vi "MoveMotor.vi"(7 "Position Mode (Absolute)":T1(ring), 8 "error in (no error)":errorcluster, 9 "Target Position (0)":i32, 10 "Axis or Vector Space":u16(ring)=1 items=["Axis 1"=1, "Axis 2"=2, "Axis 3"=3, "Axis 4"=4, "Axis 5"=5, "Axis 6"=6, "Axis 7"=7, "Axis 8"=8, "Vector Space 1"=17, "Vector Space 2"=18, "Vector Space 3"=19, "Vector Space 4"=20], 11 "Motion Bd ID":u8=1 min=1 max=32 step=1) -> (0 "error out":errorcluster, 2 "Resource Output":u16(ring) items=["Axis Control"=0, "Axis 1"=1, "Axis 2"=2, "Axis 3"=3, "Axis 4"=4, "Axis 5"=5, "Axis 6"=6, "Axis 7"=7, "Axis 8"=8, "Vector Space Control"=16, "Vector Space 1"=17, "Vector Space 2"=18, "Vector Space 3"=19, "Vector Space 4"=20, "Encoder Control"=32, "Encoder 1"=33, "Encoder 2"=34, "Encoder 3"=35, "Encoder 4"=36, "Encoder 5"=37, "Encoder 6"=38, "Encoder 7"=39, "Encoder 8"=40, "DAC Channel 1"=49, "DAC Channel 2"=50, "DAC Channel 3"=51, "DAC Channel 4"=52, "DAC Channel 5"=53, "DAC Channel 6"=54, "DAC Channel 7"=55, "DAC Channel 8"=56, "Stepper Output 1"=65, "Stepper Output 2"=66, "Stepper Output 3"=67, "Stepper Output 4"=68, "Stepper Output 5"=69, "Stepper Output 6"=70, "Stepper Output 7"=71, "Stepper Output 8"=72, "ADC Channel 1"=81, "ADC Channel 2"=82, "ADC Channel 3"=83, "ADC Channel 4"=84, "ADC Channel 5"=85, "ADC Channel 6"=86, "ADC Channel 7"=87, "ADC Channel 8"=88], 3 "Bd ID Out":u8)   [LabVIEW 2022 SP3]
uses:
  <vilib>/Motion/FlexMotion/FunctionsVIs/StartStopMotion.llb/Start Motion (8 axes).flx
  <vilib>/Motion/FlexMotion/FunctionsVIs/Trajectory.llb/Check Move Complete Status (8 axes).flx
panel:
  in  "Strict Positioning":bool
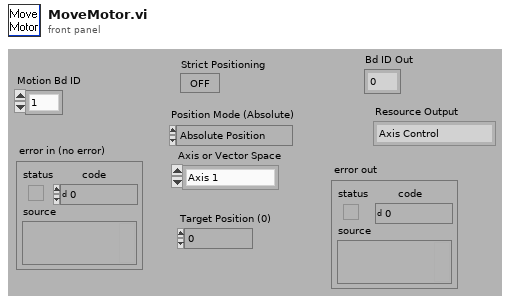
[diagram p1: front panel]
types:
  T1 = enum16{"Absolute Position", "Relative Position", "Velocity", "Relative to Cap Pos", "Modulus Position", "Absolute Contouring", "Relative Contouring"}
  T2 = typedef "Resource Out (Enum).flx" = u16
  T3 = typedef "Bd Id Out" = u8
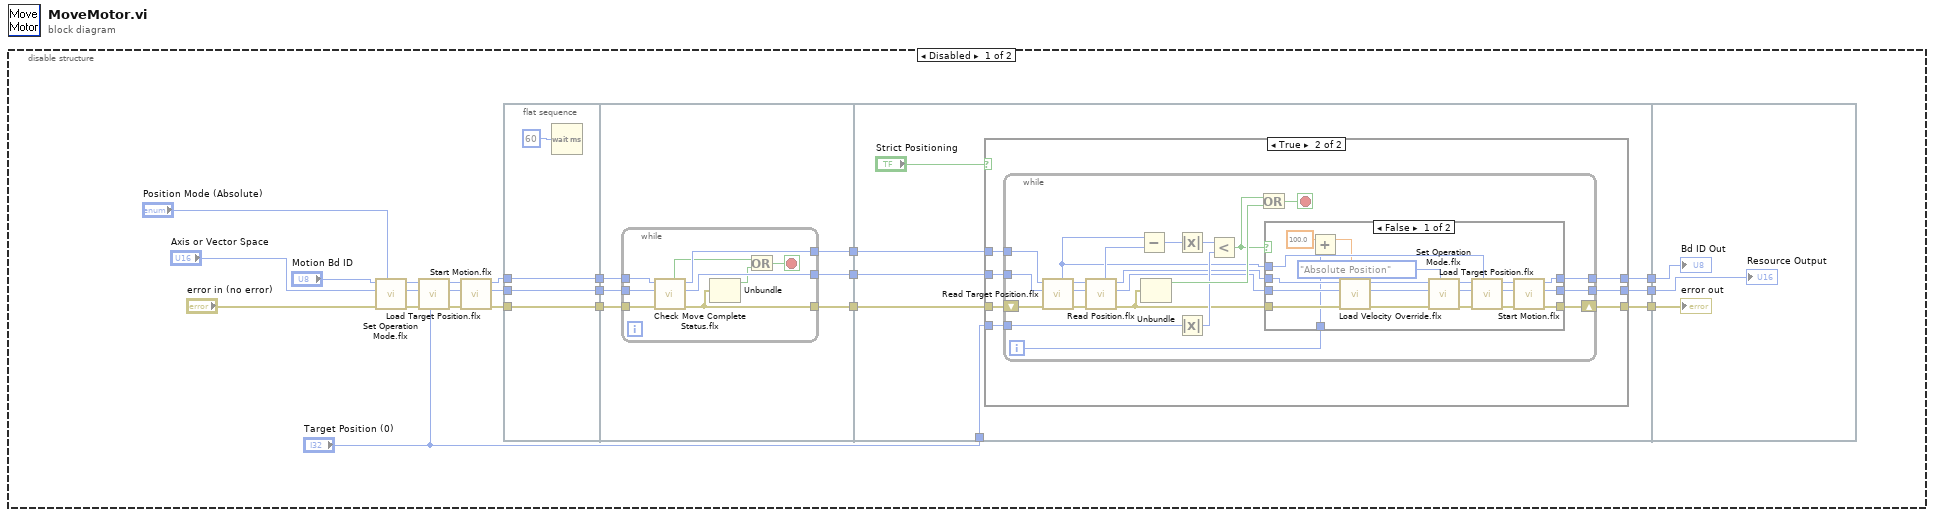
[diagram p0: block diagram]
diagram:
  n1 = disable-structure shown="Disabled" {
    frame Disabled {
      n2 = call <vilib>:"Set Operation Mode.flx"("Position Mode (Absolute)"="Position Mode (Absolute)", "error in (no error)"="error in (no error)", "Axis or Vector Space"="Axis or Vector Space", "Board ID"="Motion Bd ID") -> ("error out"=w10:errorcluster, "Resource Output"=w7:T2, "Bd ID Out"=w14:T3)  [unwired: 2 out]
      n3 = call <vilib>:"Load Target Position.flx"("Target Position (0)"="Target Position (0)", "error in (no error)"=w10, "Axis"=w7, "Board ID"=w14) -> ("error out"=w9:errorcluster, "Resource Output"=w6:T2, "Bd ID Out"=w13:T3)  [unwired: 3 out]
      n4 = call-poly <vilib>:"Start Motion.flx"("error in (no error)"=w9, "Axis or Vector Space"=w6, "Board ID"=w13) -> ("error out"=w4:errorcluster, "Resource Output"=w2:T2, "Bd ID Out"=w5:T3)  [unwired: 1 in, 2 out]
      n5 = flat-sequence {
        tunnel: w4 -> [w25]
        tunnel: w2 -> [w26]
        tunnel: w5 -> [w27]
        tunnel: [w27] -> w23
        tunnel: [w26] -> w22
        tunnel: [w25] -> w21
        tunnel: w23 -> [w33]
        tunnel: w22 -> [w32]
        tunnel: w21 -> [w31]
        tunnel: [w30] -> w20
        tunnel: [w29] -> w19
        tunnel: [w28] -> w18
        tunnel: w20 -> [w45]
        tunnel: [w44] -> w17
        tunnel: w19 -> [w48]
        tunnel: [w47] -> w16
        tunnel: w18 -> [w50]
        tunnel: [w49] -> w15
        tunnel: "Target Position (0)" -> [w43]
        tunnel: w17 -> [w108]
        tunnel: w16 -> [w107]
        tunnel: w15 -> [w106]
        frame #0 {
          n6 = Wait (ms)(milliseconds to wait=60) -> ()  [unwired: 1 out]
        }
        frame #1 {
          n7 = while {
            tunnel: w33 -> [w42]
            tunnel: w32 -> [w41]
            tunnel: w31 -> [w40]
            tunnel: [w37] -> w30
            tunnel: [w39] -> w29
            tunnel: [w38] -> w28
            stop <- w34 stop-if-true
            n8 = call-poly <vilib>:"Check Move Complete Status.flx"("error in (no error)"=w40, "Axis or Vector Space"=w41, "Board ID"=w42) -> ("error out"=w37:errorcluster, "Resource Output"=w39:T2, "Bd ID Out"=w38:T3, "Move Complete"=w35:bool)  [unwired: 1 in, 2 out]
            n9 = Unbundle(w37) -> ("status"=w36:bool)  [unwired: 2 out]
            n10 = Or(x=w35, y=w36) -> (x .or. y?=w34:bool)
          }
        }
        frame #2 {
          n11 = case shown="True" "Strict Positioning" {
            tunnel: w50 -> [w53 w60]
            tunnel: [w53 w59] -> w49
            tunnel: w48 -> [w52 w58]
            tunnel: [w52 w55] -> w47
            tunnel: w45 -> [w51 w57]
            tunnel: [w51 w54] -> w44
            tunnel: w43 -> [_ w56]
            frame False {
            }
            frame True {
              n12 = while {
                tunnel: w60 -> [w71]
                tunnel: [w68] -> w59
                tunnel: w58 -> [w70]
                tunnel: w56 -> [w76]
                tunnel: [w66] -> w55
                shift-right: [w63] -> w54
                shift-left: w57 -> [w80]
                i -> [w61]
                stop <- w77 stop-if-true
                n13 = call <vilib>:"Read Target Position.flx"("error in (no error)"=w80, "Axis"=w70, "Board ID"=w71) -> ("error out"=w79:errorcluster, "Resource Output"=w81:T2, "Bd ID Out"=w82:T3, "Target Position"=w62:i32)  [unwired: 3 in]
                n14 = call <vilib>:"Read Position.flx"("error in (no error)"=w79, "Axis"=w81, "Board ID"=w82) -> ("error out"=w64:errorcluster, "Resource Output"=w69:T2, "Bd ID Out"=w67:T3, "Position"=w65:i32)  [unwired: 3 in]
                n15 = Subtract(x=w62, y=w65) -> (x-y=w75:i32)
                n16 = Unbundle(w64) -> ("status"=w78:bool)  [unwired: 2 out]
                n17 = Absolute Value(x=w75) -> (abs(x)=w74:i32)
                n18 = Absolute Value(x=w76) -> (abs(x)=w73:i32)
                n19 = Less?(x=w74, y=w73) -> (x < y?=w72:bool)
                n20 = Or(x=w72, y=w78) -> (x .or. y?=w77:bool)
                n21 = case shown="False" w72 {
                  tunnel: w67 -> [w86 w105]
                  tunnel: w69 -> [w87 w104]
                  tunnel: [w98 w105] -> w68
                  tunnel: [w97 w104] -> w66
                  tunnel: w62 -> [w96 _]
                  tunnel: w64 -> [w91 w103]
                  tunnel: [w92 w103] -> w63
                  tunnel: w61 -> [w83 _]
                  frame False {
                    n22 = Add(x=sgl 100.0 ("Override  Percentage (100%)"), y=w83) -> (x+y=w84:sgl)
                    n23 = call <vilib>:"Load Velocity Override.flx"("Override  Percentage (100%)"=w84, "error in (no error)"=w91, "Axis or Vector Space"=w87, "Board ID"=w86) -> ("error out"=w90:errorcluster, "Resource Output"=w88:T2, "Bd ID Out"=w89:T3)  [unwired: 3 in]
                    n24 = call <vilib>:"Set Operation Mode.flx"("Position Mode (Absolute)"=T1."Absolute Position", "error in (no error)"=w90, "Axis or Vector Space"=w88, "Board ID"=w89) -> ("error out"=w94:errorcluster, "Resource Output"=w99:T2, "Bd ID Out"=w102:T3)  [unwired: 2 out]
                    n25 = call <vilib>:"Load Target Position.flx"("Target Position (0)"=w96, "error in (no error)"=w94, "Axis"=w99, "Board ID"=w102) -> ("error out"=w93:errorcluster, "Resource Output"=w100:T2, "Bd ID Out"=w101:T3)  [unwired: 3 out]
                    n26 = call-poly <vilib>:"Start Motion.flx"("error in (no error)"=w93, "Axis or Vector Space"=w100, "Board ID"=w101) -> ("error out"=w92:errorcluster, "Resource Output"=w97:T2, "Bd ID Out"=w98:T3)  [unwired: 1 in, 2 out]
                  }
                  frame True {
                  }
                }
              }
            }
          }
        }
        frame #3 {
          "error out" <- w108
          "Resource Output" <- w107
          "Bd ID Out" <- w106
        }
      }
    }
    frame Enabled {
    }
  }
